vi "Convert Raw Queue DAQ Data to Waveforms.vi"(7 "Data Rate 9215 (S/s)":dbl=1200000.0 format="%#.6p", 8 "error in":errorcluster, 9 "Signal scaling":T3[](array[typedef]), 10 "RawDAQData in":T4, 11 "Data Rate 9775(S/s)":dbl=3.0 format="%#.6p") -> (0 "error out":errorcluster, 2 "InverterWaveforms out":T1)   [LabVIEW 2019, in "Main.lvclass"]
doc: "Developed by Kevin Thompson\nkevin@thompsonengineering.net\n\nCopyright 2020\nThompson Engineering, LLC"
uses:
  Main.lvclass
  Common/DataTypes/RawDAQData--cluster.ctl
  Common/DataTypes/RawChannelData--cluster.ctl
  subvis/DataTypes/Gain control.ctl
  Common/DataTypes/InverterWaveforms--cluster.ctl
  Common/DataTypes/ChannelWaveforms--cluster.ctl
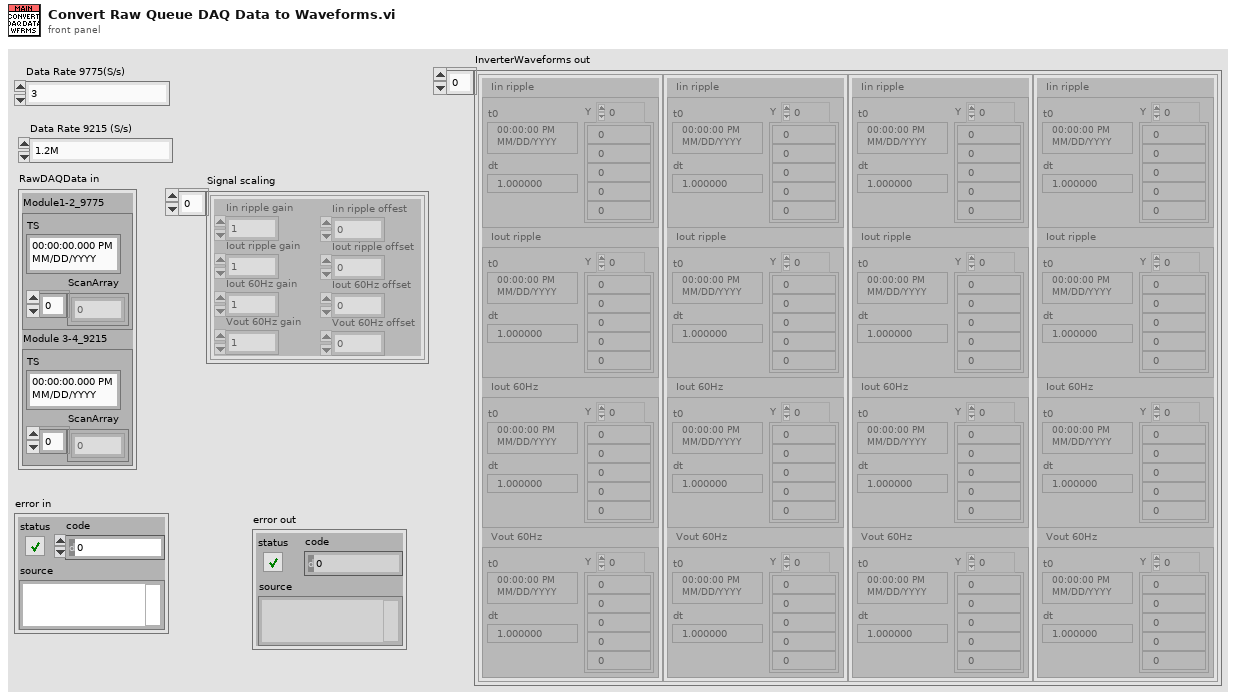
[diagram p1: front panel]
types:
  T1 = typedef "InverterWaveforms--cluster.ctl" = T2[]
  T2 = typedef "ChannelWaveforms--cluster.ctl" = cluster{"Iin ripple ":waveform(dbl), "Iout ripple ":waveform(dbl), "Iout 60Hz":waveform(dbl), "Vout 60Hz":waveform(dbl)}
  T3 = typedef "Main.lvclass/Gain control.ctl" = cluster{"Iin ripple gain":dbl, "Iout ripple gain":dbl, "Iout 60Hz gain ":dbl, "Vout 60Hz gain ":dbl, "Iin ripple offest":dbl, "Iout ripple offset":dbl, "Iout 60Hz offset":dbl, "Vout 60Hz offset":dbl}
  T4 = typedef "RawDAQData--cluster.ctl" = cluster{"Module1-2_9775":T5, "Module 3-4_9215":T5}
  T5 = typedef "RawChannelData--cluster.ctl" = cluster{"TS":timestamp, "ScanArray":dbl[]}
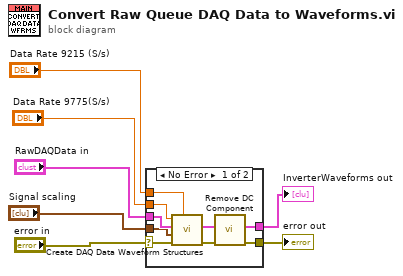
[diagram p0: block diagram]
diagram:
  n1 = case shown="No Error" "error in" {
    selector: "error in" -> [w9 w17]
    tunnel: "RawDAQData in" -> [w16 _]
    tunnel: "Signal scaling" -> [w13 _]
    tunnel: "Data Rate 9215 (S/s)" -> [w12 _]
    tunnel: [w11 _] -> w4
    tunnel: [w10 w17] -> w3
    tunnel: "Data Rate 9775(S/s)" -> [w8 _]
    frame No Error {
      n2 = call "Create DAQ Data Waveform Structures.vi"("Data Rate 9215 (S/s)"=w12, "error in"=w9, "Signal scaling"=w13, "RawDAQData in"=w16, "Data Rate 9775(S/s)"=w8) -> ("error out"=w14:errorcluster, "InverterWaveforms"=w15:T1)  [unwired: 5 in]
      n3 = call "Remove DC Component.vi"("error in"=w14, "InverterWaveforms"=w15) -> ("error out"=w10:errorcluster, "InverterWaveforms out"=w11:T1)  [unwired: 8 in]
    }
    frame Error {
    }
  }
  "error out" <- w3
  "InverterWaveforms out" <- w4
